vi "Get Attributes by Type.vi"(6 "Recurse Up List (Default=True)":bool=TRUE, 7 "Test ID":string, 8 "error in (no error)":errorcluster, 9 "Type":variant, 11 "Test Executive in":refnum<class "Test Executive.lvclass">) -> (0 "error out":errorcluster, 1 "Names":string[](array[string]), 2 "IDs":string[](array[string]), 3 "Test Executive out":refnum<class "Test Executive.lvclass">, 4 "Attributes":variant[](array[variant]))   [LabVIEW 2020, in "Test Executive.lvlib" / "Test Executive.lvclass"]
uses:
  <vilib>/gpm_packages/@cs/test-executive/Source/Test Executive/TestExecutive/Test Executive.lvclass
  <vilib>/gpm_packages/@cs/test-executive/Source/Test Executive/TestExecutive/Test Executive.lvclass/Test Executive.ctl
  7b3bf7b6-e7f3-487d-a154-e2e5367de7d1.vi
  <vilib>/Utility/error.llb/Clear Errors.vi
  <vilib>/gpm_packages/@cs/linked-list/Source/Linked List/ILinkedList/ILinked List.lvclass
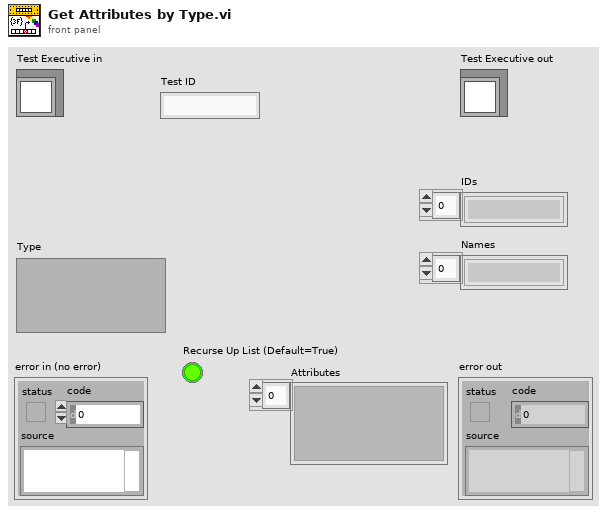
[diagram p1: front panel]
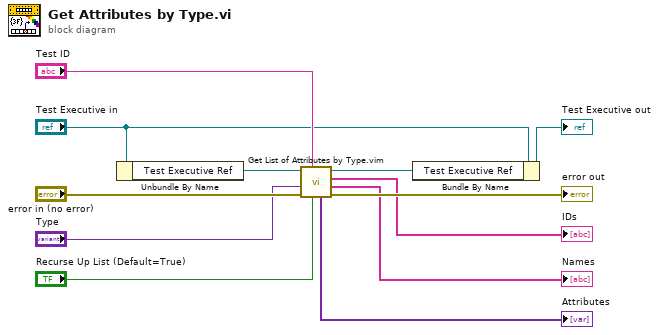
[diagram p0: block diagram]
diagram:
  n1 = Unbundle By Name("Test Executive in") -> ("Test Executive Ref"=w12:refnum<data-value>)
  n2 = call "Get List of Attributes by Type.vim"("Recurse Up List (Default=True)"="Recurse Up List (Default=True)", "Linked List ID"="Test ID", "error in (no error)"="error in (no error)", "Type"="Type", "Linked List Ref"=w12) -> ("error out"=→"error out":errorcluster, "Names"=→"Names":string[], "IDs"=→"IDs":string[], "Linked List Ref out"=w3:refnum<data-value>, "Attributes"=→"Attributes":variant[])  [unwired: 2 in]
  n3 = Bundle By Name(cluster="Test Executive in", "Test Executive Ref"=w3) -> (→"Test Executive out":refnum<class "Test Executive.lvclass">)
